vi "Read Bit.vi"(8 "error in (no error)":errorcluster, 11 "Low Speed in":refnum<class "Low Speed.lvclass">) -> (0 "error out":errorcluster, 3 "Low Speed out":refnum<class "Low Speed.lvclass">)   [LabVIEW 2020, in "Low Speed.lvclass"]
uses:
  Low Speed.lvclass
  C:/Users/kaiser.asan/OneDrive - SolitonTechnologies/LabVIEW/29.SDLC - I2C Driver/I2C Module/I2C Controller Module/Class/Transmission Mode/Parent/TX Speed.lvclass
  Low Speed.lvclass/Low Speed.ctl
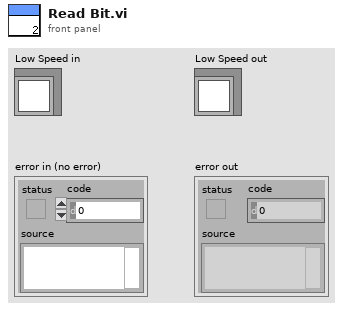
[diagram p1: front panel]
types:
  T1 = typedef "I2C Controller Lib.lvlib/Timing Parameters Cluster.ctl" = cluster{"f_SCL(KHz)":u32, "t_HIGH (ns)":u32, "t_LOW (ns)":u32, "t_SU;STA (ns)":u32, "t_HD;STA (ns)":u32, "t_SU;DAT (ns)":u32, "t_HD;DAT (ns)":u32, "t_SU;STO (ns)":u32, "t_BUF (ns)":u32}
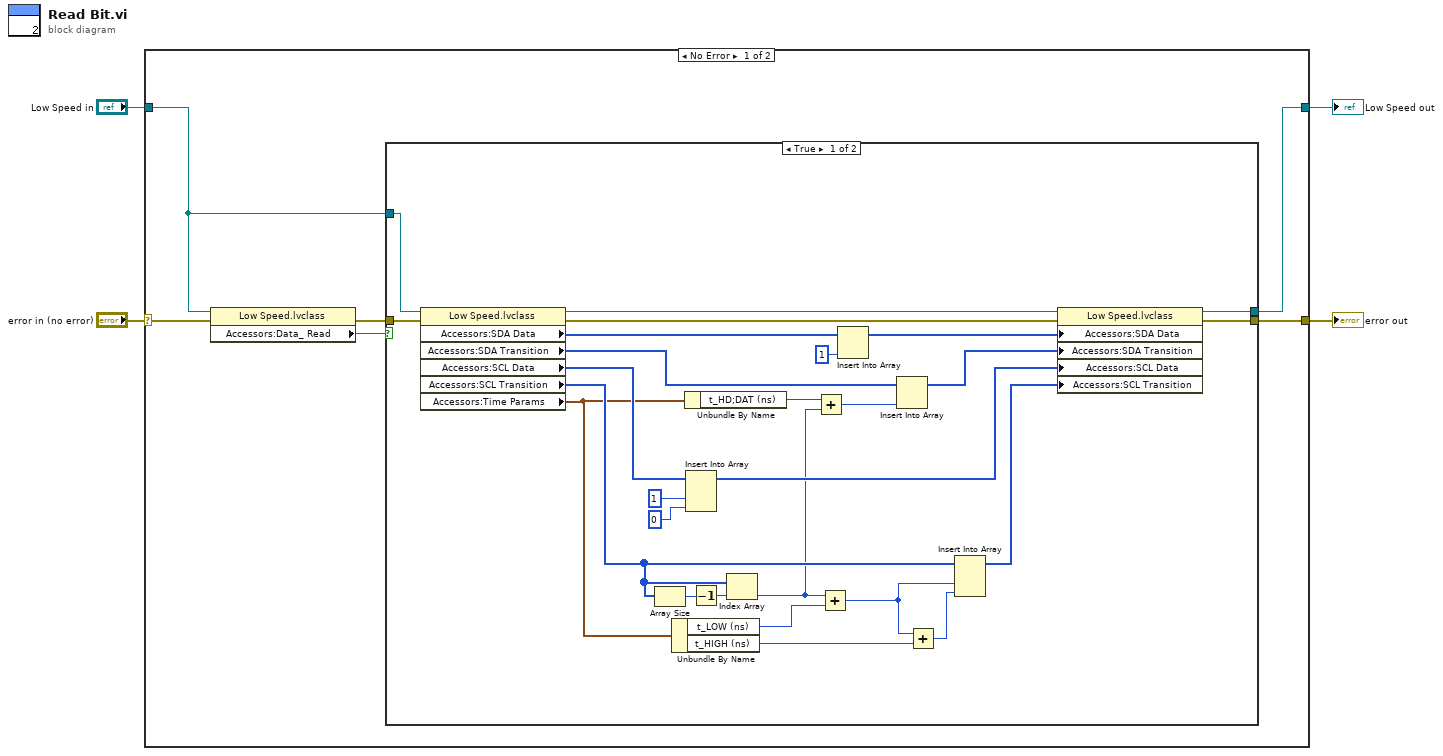
[diagram p0: block diagram]
diagram:
  n1 = case shown="No Error" "error in (no error)" {
    selector: "error in (no error)" -> [w10 w41]
    tunnel: [w5 w40] -> w4
    tunnel: "Low Speed in" -> [w6 w40]
    tunnel: [w8 w41] -> w2
    frame No Error {
      n2 = property class="Low Speed.lvclass"(reference=w6, error in=w10) -> (error out=w7:errorcluster, "Accessors:Data_ Read"=w9:bool)  [unwired: 1 out]
      n3 = case shown="True" w9 {
        tunnel: [w32 w38] -> w8
        tunnel: w7 -> [w37 w38]
        tunnel: w6 -> [w35 w39]
        tunnel: [w30 w39] -> w5
        frame True {
          n4 = property class="Low Speed.lvclass"(reference=w35, error in=w37) -> (reference out=w31:refnum<class "Low Speed.lvclass">, error out=w36:errorcluster, "Accessors:SDA Data"=w19:u8[], "Accessors:SDA Transition"=w14:u32[], "Accessors:SCL Data"=w29:u8[], "Accessors:SCL Transition"=w21:u32[], "Accessors:Time Params"=w15:T1)
          n5 = Array Size(array=w21) -> (size(s)=w27:i32)
          n6 = Unbundle By Name(w15) -> ("t_LOW (ns)"=w25:u32, "t_HIGH (ns)"=w24:u32)
          n7 = Unbundle By Name(w15) -> ("t_HD;DAT (ns)"=w12:u32)
          n8 = Insert Into Array(array=w29, new element #1=u8 1 ("new element/subarray"), new element #2=u8 0 ("new element/subarray")) -> (w28:u8[])  [unwired: 1 in]
          n9 = Decrement(x=w27) -> (x-1=w26:i32)
          n10 = Index Array(array=w21, index=w26) -> (element=w11:u32)
          n11 = Add(x=w12, y=w11) -> (x+y=w16:u32)
          n12 = Add(x=w11, y=w25) -> (x+y=w22:u32)
          n13 = Insert Into Array(array=w19, new element=u8 1 ("new element/subarray")) -> (w18:u8[])  [unwired: 1 in]
          n14 = Insert Into Array(array=w14, new element=w16) -> (w13:u32[])  [unwired: 1 in]
          n15 = Add(x=w22, y=w24) -> (x+y=w23:u32)
          n16 = Insert Into Array(array=w21, new element #1=w22, new element #2=w23) -> (w20:u32[])  [unwired: 1 in]
          n17 = property class="Low Speed.lvclass"(reference=w31, error in=w36, "Accessors:SDA Data"=w18, "Accessors:SDA Transition"=w13, "Accessors:SCL Data"=w28, "Accessors:SCL Transition"=w20) -> (reference out=w30:refnum<class "Low Speed.lvclass">, error out=w32:errorcluster)
        }
        frame False {
        }
      }
    }
    frame Error {
    }
  }
  "error out" <- w2
  "Low Speed out" <- w4
